vi "CreateLVINILocalHostKey.vi"   [LabVIEW 2021]
uses:
  <vilib>/Utility/config.llb/Write Key (String).vi
  <vilib>/Wiresmith Technology/G CLI/CLI Class/CLI.lvclass
  <vilib>/Utility/config.llb/NI_LVConfig.lvlib
types:
  T1 = enum32{"Invalid", "Standard", "Closed", "Hidden", "Minimized", "Maximized"}
  T2 = typedef "NI_LVConfig.lvlib/Config Data RefNum.ctl" = refnum<k1>
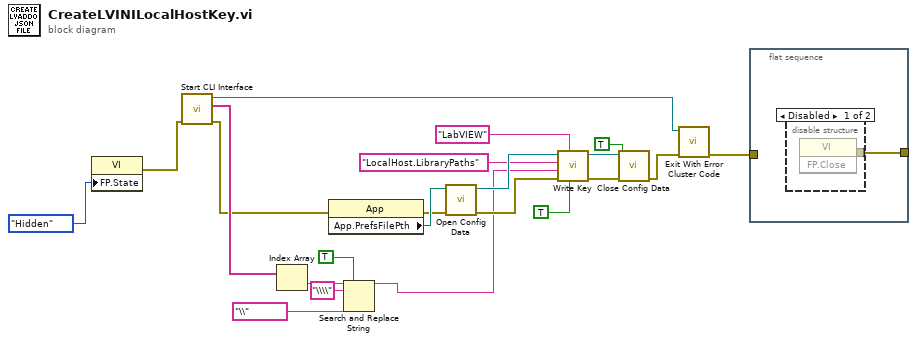
[diagram p0: block diagram]
diagram:
  n1 = property class="VI"("FP.State"=T1."Hidden" ("Front Panel Window:State")) -> (error out=w21:errorcluster)  [unwired: 2 in, 1 out]
  n2 = call <vilib>:"Start CLI Interface.vi"("error in (no error)"=w21) -> ("error out"=w4:errorcluster, "Custom Parameters"=w9:string[], "CLI out"=w19:refnum<class "CLI.lvclass">)  [unwired: 7 in, 1 out]
  n3 = Index Array(array=w9) -> (element=w8:string)  [unwired: 1 in]
  n4 = property class="App"(error in=w4) -> (error out=w13:errorcluster, "App.PrefsFilePth"=w18:path)  [unwired: 1 in, 1 out]
  n5 = Search and Replace String(replace all?=TRUE ("replace all? (F)"), input string=w8, search string="\\\\", replace string="\\" ("replace string (\"\")")) -> (result string=w3:string)  [unwired: 4 in, 3 out]
  n6 = call <vilib>:"Open Config Data.vi"("error in (no error)"=w13, "configuration file path"=w18) -> ("error out"=w14:errorcluster, "refnum"=w17:T2)  [unwired: 7 in, 1 out]
  n7 = call-poly <vilib>:"Write Key.vi"("write raw string? (F)"=TRUE, "section"="LabVIEW", "error in (no error)"=w14, "value"=w3, "key"="LocalHost.LibraryPaths", "refnum"=w17) -> ("error out"=w11:errorcluster, "refnum out"=w10:T2)  [unwired: 3 in, 1 out]
  n8 = call <vilib>:"Close Config Data.vi"("error in (no error)"=w11, "write file if changed (T)"=TRUE, "refnum"=w10) -> ("error out"=w12:errorcluster)  [unwired: 7 in, 1 out]
  n9 = call <vilib>:"Exit With Error Cluster Code.vi"("error in (no error)"=w12, "CLI in"=w19) -> ("error out"=w20:errorcluster)  [unwired: 9 in]
  n10 = flat-sequence {
    tunnel: [w23] -> _
    tunnel: w20 -> [_]
    frame #0 {
      n11 = disable-structure shown="Disabled" {
        disable-tunnel: [w24 _] -> w23
        frame Disabled {
          n12 = invoke class="VI" method="FP.Close"() -> (error out=w24:errorcluster)  [unwired: 3 in, 2 out]
        }
        frame Enabled {
        }
      }
    }
  }
